vi "ThermoV_ControlSweep_NoMean_160801.vi"() -> ()   [LabVIEW 2013]
panel:
  out "subarray":dbl[](array[numeric])
  out "Array":dbl[](array[numeric])
  in  "Operate HVpp\nOutput Timer":bool caption="Reset"
  out "modular 13":dbl
  in  "Number of seconds for \neach HVpp case state":dbl=30.0
  out "Elapsed Time (s)":dbl
  out "DC Value":dbl[](array[numeric]) format="%#.6f"
  in  "Saving Avg?":bool
  in  "Filename":path=path "trial_1.lvm"
  in  "STOP":bool
  in  "Save Waveform":bool
  out "Peak2Peak V":dbl[](array[numeric])
  out "Waveform Chart":dynamicdata(graph)
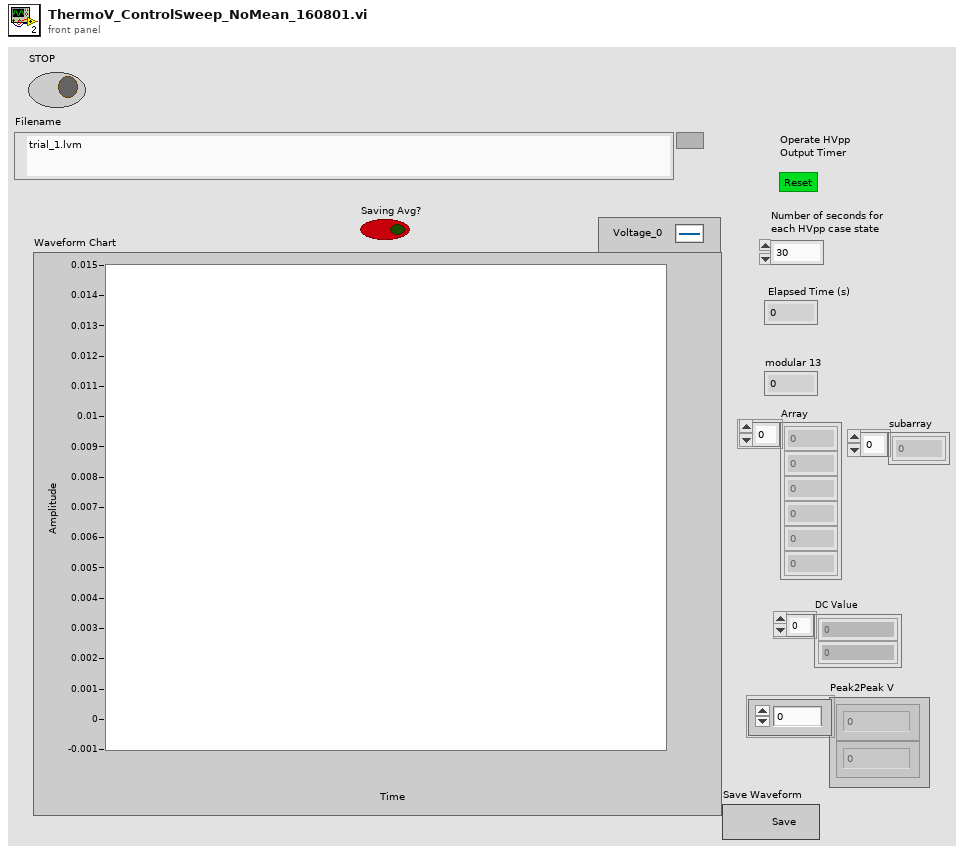
[diagram p1: front panel]
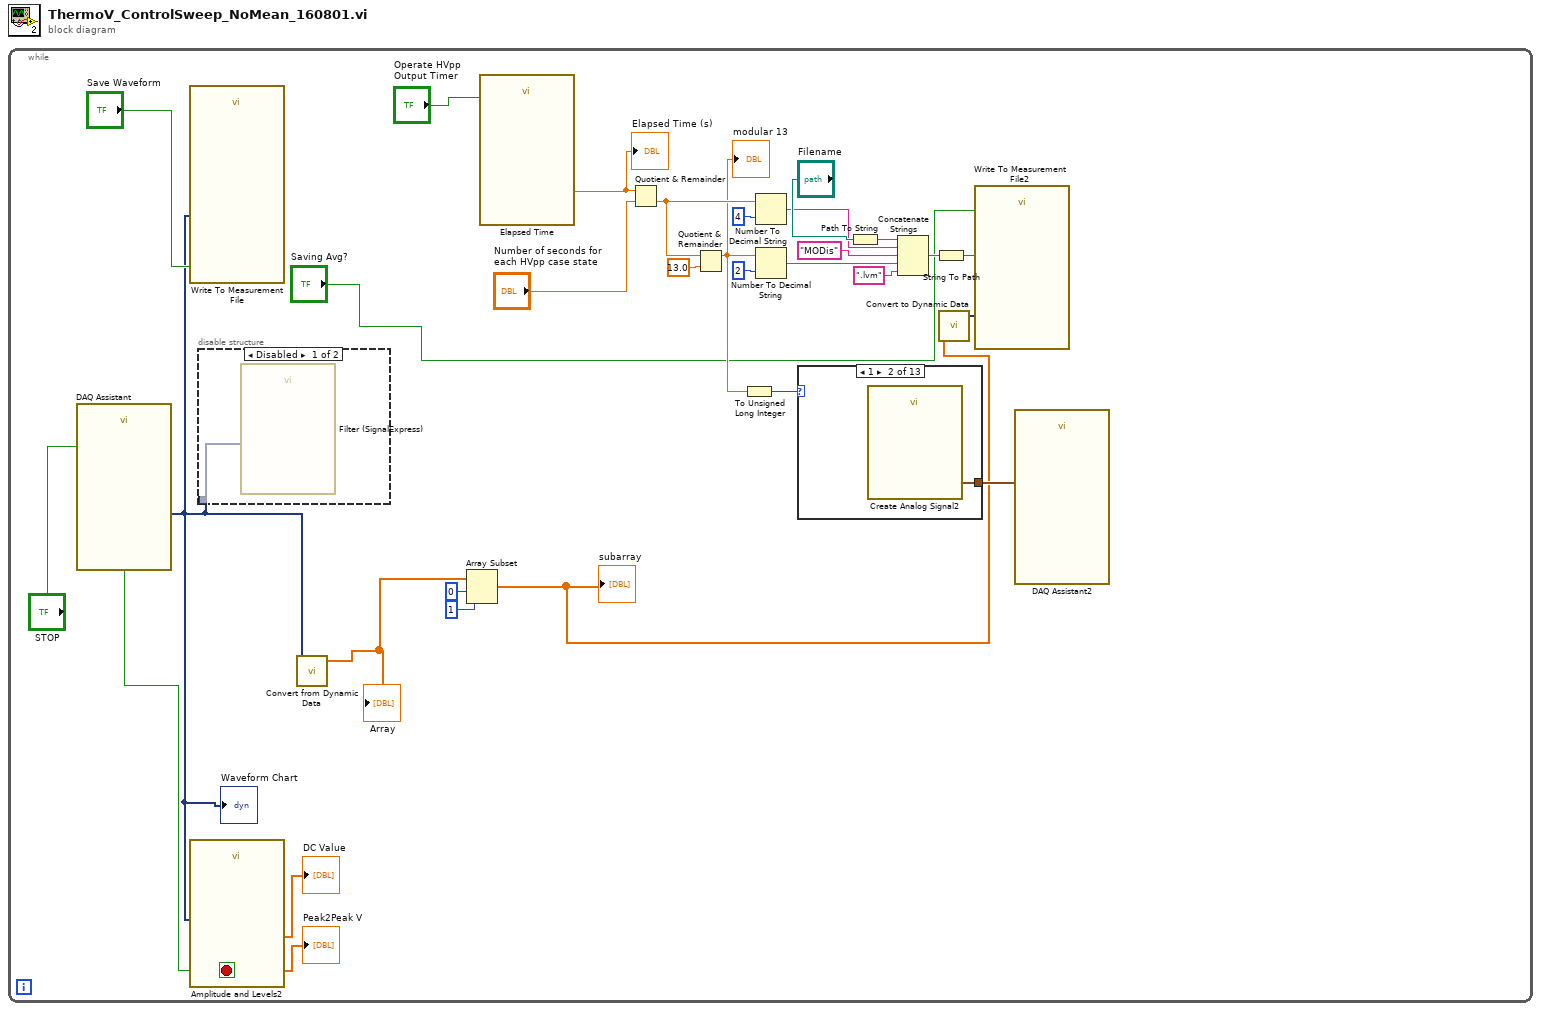
[diagram p0: block diagram]
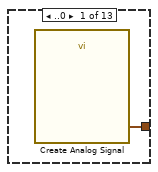
[diagram p3: hidden frame]
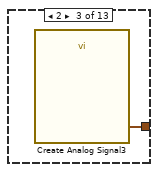
[diagram p4: hidden frame]
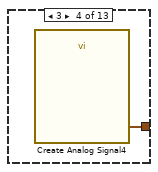
[diagram p5: hidden frame]
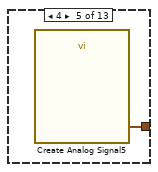
[diagram p6: hidden frame]
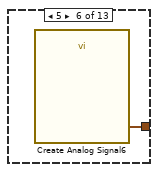
[diagram p7: hidden frame]
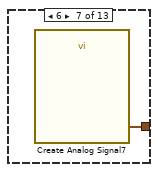
[diagram p8: hidden frame]
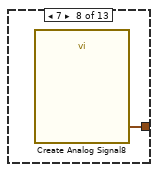
[diagram p9: hidden frame]
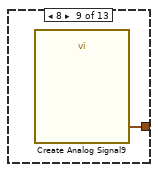
[diagram p10: hidden frame]
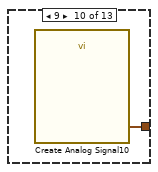
[diagram p11: hidden frame]
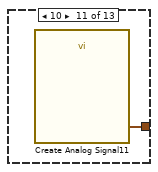
[diagram p12: hidden frame]
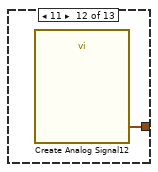
[diagram p13: hidden frame]
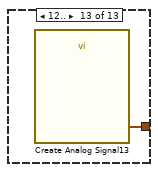
[diagram p14: hidden frame]
diagram:
  n1 = while {
    stop <- w30 stop-if-true
    n2 = call "DAQ Assistant"("stop (F)"="STOP") -> ("data"=w1:dynamicdata, "stopped"=w30:bool)  [unwired: 15 in, 2 out]
    "Waveform Chart" <- w1
    n3 = call "Write To Measurement File"("Signals"=w1, "Enable"="Save Waveform") -> ()  [unwired: 15 in, 3 out]
    n4 = call "Amplitude and Levels2"("input signals"=w1) -> ("dc"=→"DC Value":dbl[], "peak-peak"=→"Peak2Peak V":dbl[])  [unwired: 15 in, 2 out]
    n5 = disable-structure shown="Disabled" {
      disable-tunnel: w1 -> [w31 _]
      frame Disabled {
        n6 = call "Filter (SignalExpress)"("input signal"=w31) -> ()  [unwired: 17 in, 2 out]
      }
      frame Enabled {
      }
    }
    n7 = call "Convert from Dynamic Data"("Dynamic Data Type"=w1) -> ("Array"=w6:dbl[])  [unwired: 3 in]
    "Array" <- w6
    n8 = Array Subset(array=w6, index=0, length=1) -> (w3:dbl[])
    "subarray" <- w3
    n9 = call "Elapsed Time"("Reset"="Operate HVpp\nOutput Timer") -> ("Elapsed Time (s)"=w23:dbl)  [unwired: 11 in, 7 out]
    "Elapsed Time (s)" <- w23
    n10 = Quotient & Remainder(x=w23, y="Number of seconds for \neach HVpp case state") -> (floor(x/y)=w15:dbl)  [unwired: 1 out]
    n11 = Quotient & Remainder(x=w15, y=13.0) -> (x-y*floor(x/y)=w10:dbl)  [unwired: 1 out]
    "modular 13" <- w10
    n12 = To Unsigned Long Integer(number=w10) -> (unsigned 32bit integer=w24:u32)
    n13 = Number To Decimal String(number=w15, width (-)=i16 4) -> (decimal integer string=w14:string)
    n14 = Number To Decimal String(number=w10, width (-)=i16 2) -> (decimal integer string=w9:string)
    n15 = case shown="1" w24 {
      tunnel: [w32 w33 w34 w35 w36 w37 w38 w39 w40 w41 w42 w43 w44] -> w25
      frame ..0 {
        n16 = call "Create Analog Signal"() -> ("sine wave"=w32:waveform(dbl))  [unwired: 18 in, 1 out]
      }
      frame 1 {
        n17 = call "Create Analog Signal2"() -> ("sine wave"=w33:waveform(dbl))  [unwired: 18 in, 1 out]
      }
      frame 2 {
        n18 = call "Create Analog Signal3"() -> ("sine wave"=w34:waveform(dbl))  [unwired: 18 in, 1 out]
      }
      frame 3 {
        n19 = call "Create Analog Signal4"() -> ("sine wave"=w35:waveform(dbl))  [unwired: 18 in, 1 out]
      }
      frame 4 {
        n20 = call "Create Analog Signal5"() -> ("sine wave"=w36:waveform(dbl))  [unwired: 18 in, 1 out]
      }
      frame 5 {
        n21 = call "Create Analog Signal6"() -> ("sine wave"=w37:waveform(dbl))  [unwired: 18 in, 1 out]
      }
      frame 6 {
        n22 = call "Create Analog Signal7"() -> ("sine wave"=w38:waveform(dbl))  [unwired: 18 in, 1 out]
      }
      frame 7 {
        n23 = call "Create Analog Signal8"() -> ("sine wave"=w39:waveform(dbl))  [unwired: 18 in, 1 out]
      }
      frame 8 {
        n24 = call "Create Analog Signal9"() -> ("sine wave"=w40:waveform(dbl))  [unwired: 18 in, 1 out]
      }
      frame 9 {
        n25 = call "Create Analog Signal10"() -> ("sine wave"=w41:waveform(dbl))  [unwired: 18 in, 1 out]
      }
      frame 10 {
        n26 = call "Create Analog Signal11"() -> ("sine wave"=w42:waveform(dbl))  [unwired: 18 in, 1 out]
      }
      frame 11 {
        n27 = call "Create Analog Signal12"() -> ("sine wave"=w43:waveform(dbl))  [unwired: 18 in, 1 out]
      }
      frame 12.. {
        n28 = call "Create Analog Signal13"() -> ("sine wave"=w44:waveform(dbl))  [unwired: 18 in, 1 out]
      }
    }
    n29 = Path To String(path="Filename") -> (string=w17:string)
    n30 = Concatenate Strings(w17, w14, "MODis" ("string"), w9, ".lvm" ("string")) -> (w19:string)
    n31 = String To Path(string=w19) -> (path=w20:path)
    n32 = call "Convert to Dynamic Data"("Array"=w3) -> ("Dynamic Data Type"=w2:dynamicdata)  [unwired: 3 in]
    n33 = call "Write To Measurement File2"("Signals"=w2, "Enable"="Saving Avg?", "Filename"=w20) -> ()  [unwired: 14 in, 3 out]
    n34 = call "DAQ Assistant2"("data"=w25) -> ()  [unwired: 16 in, 3 out]
  }
